vi "PalmSense Initialize Hardware References.vi"(8 "error in (no error)":errorcluster, 10 "Data":variant, 11 "Hardware Resources in":T1) -> (0 "error out":errorcluster, 3 "Hardware Resources out":T1)   [LabVIEW 2020, in "PalmSens.lvlib"]
doc: "Initialize the hardware references."
uses:
  PalmSens.lvlib
  PalmSense Hardware Configuration.ctl
  <instrlib>/PalmSens SDK for LabVIEW 5.10/PalmSens/PalmSens.lvclass
  support/Message Queue/Message Cluster.ctl
  support/Message Queue/Message Queue.lvlib
panel:
  out "Array":string[](array[string])
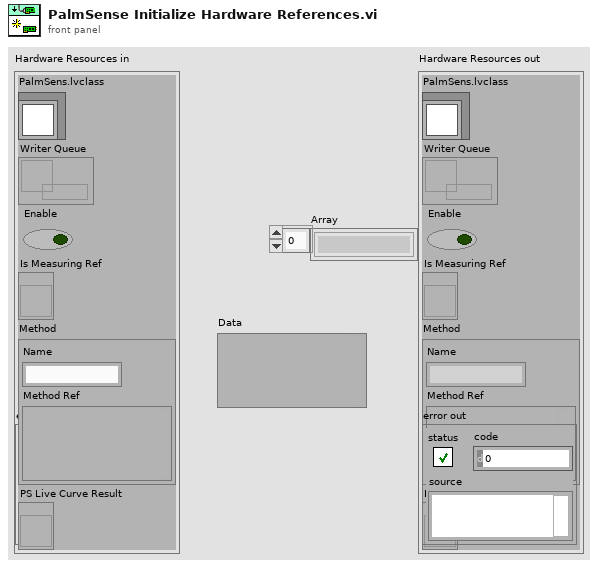
[diagram p1: front panel]
types:
  T1 = typedef "PalmSens.lvlib/PalmSense Hardware Configuration.ctl" = cluster{"PalmSens.lvclass":refnum<class "PalmSens.lvclass">, "Writer Queue":refnum<queue>, "Enable":bool, "Is Measuring Ref":refnum<vi>, "Method":cluster{"Name":string, "Method Ref":variant}, "PS Live Curve Result":refnum<vi>}
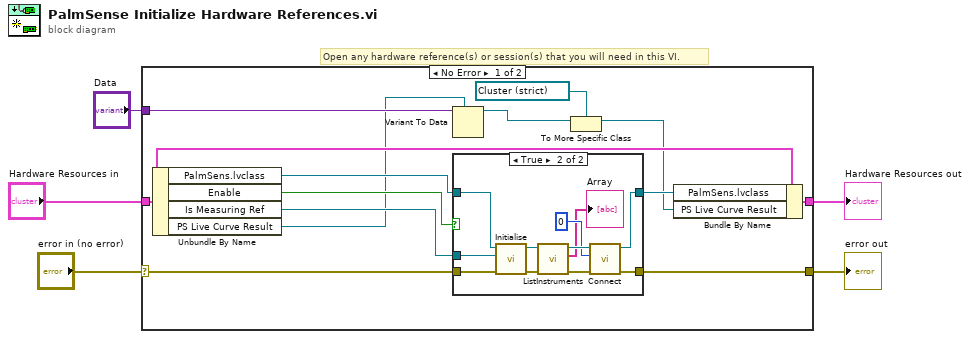
[diagram p0: block diagram]
diagram:
  # "Open any hardware reference(s) or session(s) that you will need in this VI."
  n1 = case shown="No Error" "error in (no error)" {
    selector: "error in (no error)" -> [w16 w32]
    tunnel: [w13 w32] -> w4
    tunnel: "Hardware Resources in" -> [w18 w33]
    tunnel: [w14 w33] -> w2
    tunnel: "Data" -> [w10 _]
    frame No Error {
      n2 = Unbundle By Name(w18) -> ("PalmSens.lvclass"=w17:refnum<class "PalmSens.lvclass">, "Enable"=w12:bool, "Is Measuring Ref"=w11:refnum<vi>, "PS Live Curve Result"=w9:refnum<vi>)
      n3 = Variant To Data(type=w9, Variant=w10) -> (data=w7:refnum<vi>)  [unwired: 1 in, 1 out]
      n4 = case shown="True" w12 {
        tunnel: w17 -> [w19 w31]
        tunnel: w16 -> [w20 w30]
        tunnel: [w19 w27] -> w15
        tunnel: [w20 w23] -> w13
        tunnel: w11 -> [_ w22]
        frame False {
        }
        frame True {
          n5 = call-dynamic "Initialise.vi"("error in (no error)"=w30, "Is Measuring Refnum"=w22, "PalmSens in"=w31) -> ("error out"=w26:errorcluster, "PalmSens out"=w29:refnum<class "PalmSens.lvclass">)  [unwired: 7 in]
          n6 = call-dynamic "ListInstruments.vi"("error in (no error)"=w26, "PalmSens in"=w29) -> ("error out"=w25:errorcluster, "Array"=→"Array":string[], "PalmSens out"=w28:refnum<class "PalmSens.lvclass">)  [unwired: 7 in]
          n7 = call-dynamic "Connect.vi"("error in (no error)"=w25, "Instrument Index"=0, "PalmSens in"=w28) -> ("error out"=w23:errorcluster, "PalmSens out"=w27:refnum<class "PalmSens.lvclass">)  [unwired: 7 in]
        }
      }
      n8 = To More Specific Class(target class=refnum<vi> refnum ("PS Live Curve Result"), reference=w7) -> (specific class reference=w6:refnum<vi>)  [unwired: 1 in, 1 out]
      n9 = Bundle By Name(cluster=w18, "PalmSens.lvclass"=w15, "PS Live Curve Result"=w6) -> (w14:T1)
    }
    frame Error {
    }
  }
  "Hardware Resources out" <- w2
  "error out" <- w4
